vi "Write WebSocket Data Handler.vi"(8 "error in (no error)":errorcluster, 10 "WebSocket Actor.lvlib:WebSocket Data Handler Msg.lvclass":refnum<class "WebSocket Data Handler Msg.lvclass">, 11 "WebSocket Service Actor in":refnum<class "WebSocket Service Actor.lvclass">) -> (0 "error out":errorcluster, 3 "WebSocket Service Actor out":refnum<class "WebSocket Service Actor.lvclass">)   [LabVIEW 2016, in "WebSocket Actor.lvlib" / "WebSocket Service Actor.lvclass"]
uses:
  WebSocket Service Actor.lvclass
  Abstract Messages/WebSocket Data Handler Msg/WebSocket Data Handler Msg.lvclass
  WebSocket Service Actor.lvclass/WebSocket Service Actor.ctl
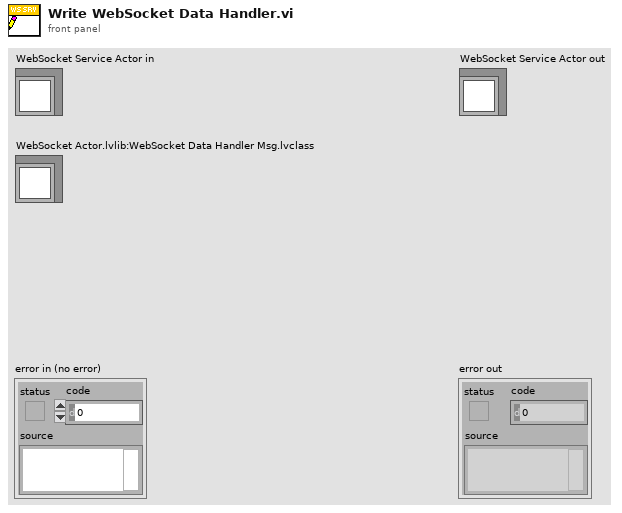
[diagram p1: front panel]
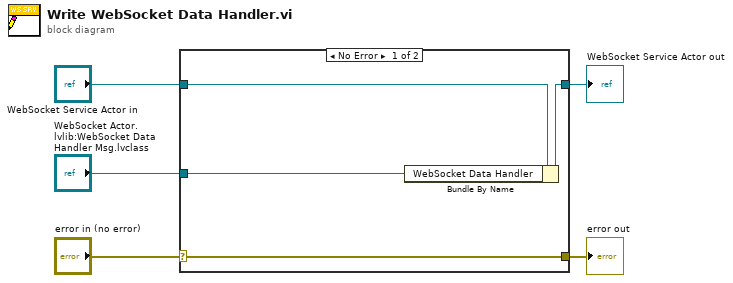
[diagram p0: block diagram]
diagram:
  n1 = case shown="No Error" "error in (no error)" {
    selector: "error in (no error)" -> [w9 w10]
    tunnel: [w9 w10] -> w4
    tunnel: [w7 w11] -> w2
    tunnel: "WebSocket Service Actor in" -> [w8 w11]
    tunnel: "WebSocket Actor.lvlib:WebSocket Data Handler Msg.lvclass" -> [w6 _]
    frame No Error {
      n2 = Bundle By Name(cluster=w8, "WebSocket Data Handler"=w6) -> (w7:refnum<class "WebSocket Service Actor.lvclass">)
    }
    frame Error {
    }
  }
  "error out" <- w4
  "WebSocket Service Actor out" <- w2
